vi "ContMotionFixPRF.vi"(0 "Offset":i32, 6 "steps between scans":sgl format="%.2f", 8 "total steps in line":i32=100, 9 "Axis":i32=1 min=1 max=4) -> (3 "Output String":string)   [LabVIEW 2022 SP3]
uses:
  -MotionRoutines/MotionGlobals.vi
panel:
  out "wait ms":i32=1
  in  "prf line":i32=3
  out "length":i32
  # "Not used anymore"
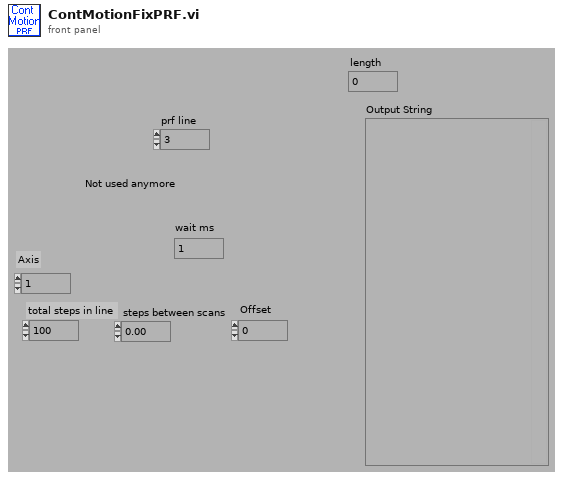
[diagram p1: front panel]
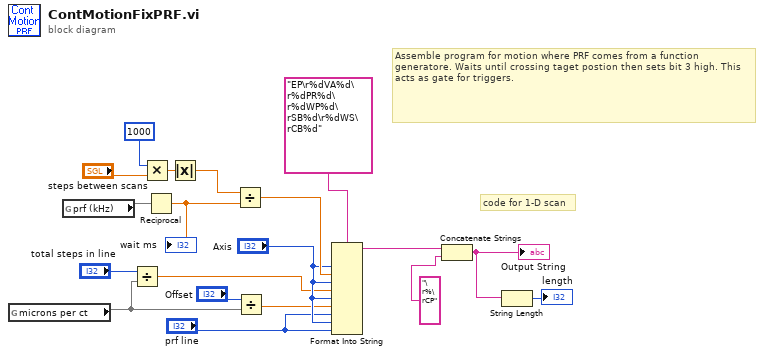
[diagram p0: block diagram]
diagram:
  # "code for 1-D scan"
  # "Assemble program for motion where PRF comes from a function generatore. Waits until crossing taget postion then sets bit 3 high. This acts as gate for triggers."
  n1 = global read "MotionGlobals.vi" "microns per ct"() -> (w2)
  n2 = global read "MotionGlobals.vi" "prf (kHz)"() -> (w8)
  n3 = Divide(x="total steps in line", y=w2) -> (x/y=w5:dbl)
  n4 = Multiply(x=1000, y="steps between scans") -> (x*y=w15:sgl)
  n5 = Reciprocal(x=w8) -> (1/x=w7:dbl)
  "wait ms" <- w7
  n6 = Absolute Value(x=w15) -> (abs(x)=w16:sgl)
  n7 = Divide(x=w16, y=w7) -> (x/y=w12:sgl)
  n8 = Divide(x="Offset", y=w2) -> (x/y=w3:dbl)
  n9 = Format Into String(format string="EP\r%dVA%d\r%dPR%d\r%dWP%d\rSB%d\r%dWS\rCB%d", "Axis", w12, "Axis", w5, "Axis", w3, "prf line", "Axis", "prf line") -> (resulting string=w11:string)  [unwired: 2 in, 1 out]
  n10 = Concatenate Strings(w11, "\r%\rCP") -> (w17:string)
  "Output String" <- w17
  n11 = String Length(string=w17) -> (length=→"length":i32)
